vi "init_measuring_devices.vi"(8 "error in (no error)":errorcluster, 11 "UI":T1) -> (0 "error out":errorcluster, 3 "UI out":T1)   [LabVIEW 2017]
uses:
  ui.ctl
  classes/dc_power_supply/DC_power_supply.lvclass
  classes/report/Report.lvclass
  ui_buttons.ctl
  types/boc_type.ctl
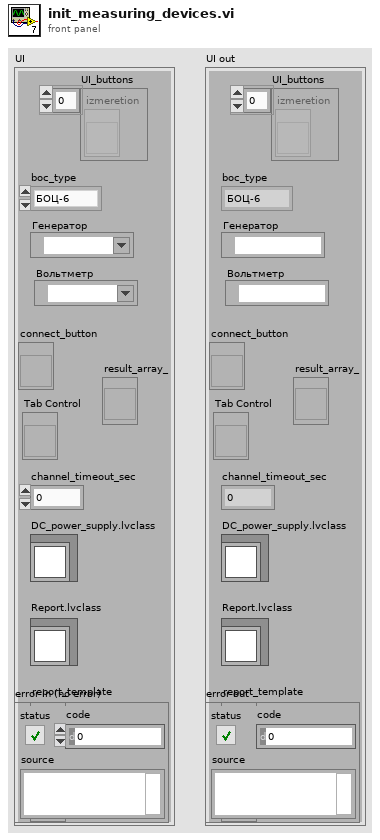
[diagram p1: front panel]
types:
  T1 = typedef "ui.ctl" = cluster{"UI_buttons":T2, "Tab Control":refnum<vi>, "connect_button":refnum<vi>, "generator":refnum<visa-resource-name>, "voltmetr":refnum<visa-resource-name>, "channel_timeout_sec":dbl, "boc_type":T3, "result_array_":refnum<vi>, "DC_power_supply.lvclass":refnum<class "DC_power_supply.lvclass">, "Report.lvclass":refnum<class "Report.lvclass">, "report_template":refnum<vi>, "report":refnum<vi>}
  T2 = typedef "ui_buttons.ctl" = refnum<vi>[]
  T3 = typedef "boc_type.ctl" = enum16{"БОЦ-6", "БОЦ-12"}
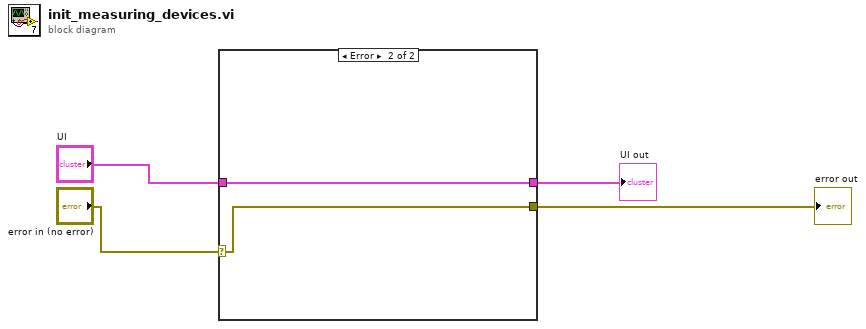
[diagram p0: block diagram]
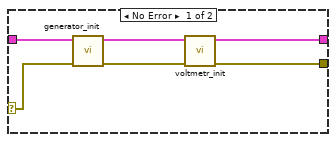
[diagram p2: hidden frame]
diagram:
  n1 = case shown="Error" "error in (no error)" {
    selector: "error in (no error)" -> [w5 w11]
    tunnel: [w10 w12] -> w4
    tunnel: [w9 w11] -> w3
    tunnel: "UI" -> [w8 w12]
    frame No Error {
      n2 = call "generator_init.vi"("error in (no error)"=w5, "UI in"=w8) -> ("error out"=w7:errorcluster, "UI out"=w6:T1)  [unwired: 8 in]
      n3 = call "voltmetr_init.vi"("error in (no error)"=w7, "UI in"=w6) -> ("error out"=w9:errorcluster, "UI out"=w10:T1)  [unwired: 8 in]
    }
    frame Error {
    }
  }
  "UI out" <- w4
  "error out" <- w3
